vi "Teleop.vi"(10 "Match Info":T1={"Autonomous Elapsed Seconds"=0.0, "TeleOp Elapsed Seconds"=0.0, "Disabled Elapsed Seconds"=0.0, "Visited Autonomous"=FALSE, "Visited TeleOp"=FALSE, "Visited Disabled"=FALSE, "Autonomous Settings"={"Autonomous Style"=enum."Independent", "VI Refnum"=refnum}}, 11 "Call Context":T2) -> ()   [LabVIEW 2014]
doc: "This VI is called for each TeleOp packet received from the DS where the robot is not disabled. It is often used to read from the joysticks and update I/O or to update setpoints for timed control loops. It should complete and return within 20 milliseconds or it may miss DS packets."
uses:
  <vilib>/Rock Robotics/WPI/DriverStation/WPI_DriverStationDerivedRobotMode.ctl
  <vilib>/Rock Robotics/WPI/DriverStation/WPI_DriverStationMatch Info.ctl
  <vilib>/Rock Robotics/WPI/Joystick/WPI_JoystickGetSetRefNum.vi
  Robot Global Data.vi
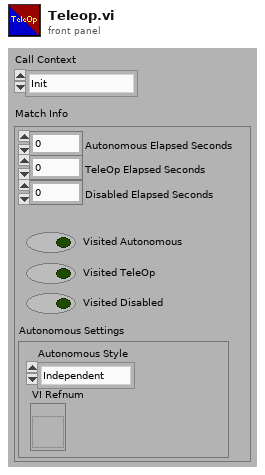
[diagram p1: front panel]
types:
  T1 = typedef "WPI_DriverStationMatch Info.ctl" = cluster{"Autonomous Elapsed Seconds":dbl, "TeleOp Elapsed Seconds":dbl, "Disabled Elapsed Seconds":dbl, "Visited Autonomous":bool, "Visited TeleOp":bool, "Visited Disabled":bool, "Autonomous Settings":cluster{"Autonomous Style":enum16{"Iterative", "Independent"}, "VI Refnum":refnum<vi>}}
  T2 = typedef "WPI_DriverStationDerivedRobotMode.ctl" = enum16{"Init", "Execute", "Stop"}
  T3 = cluster{"Initial Case":enum16{"Theta", "Arc"}, "Drive Case":enum16{"FOD", "ROD"}}
  T4 = typedef "WPI_JoystickDevRef.ctl" = cluster{"Device":T5}
  T5 = typedef "WPI_JoystickDeviceEnum.ctl" = enum16{"USB 0", "USB 1", "USB 2", "USB 3", "USB 4", "USB 5"}
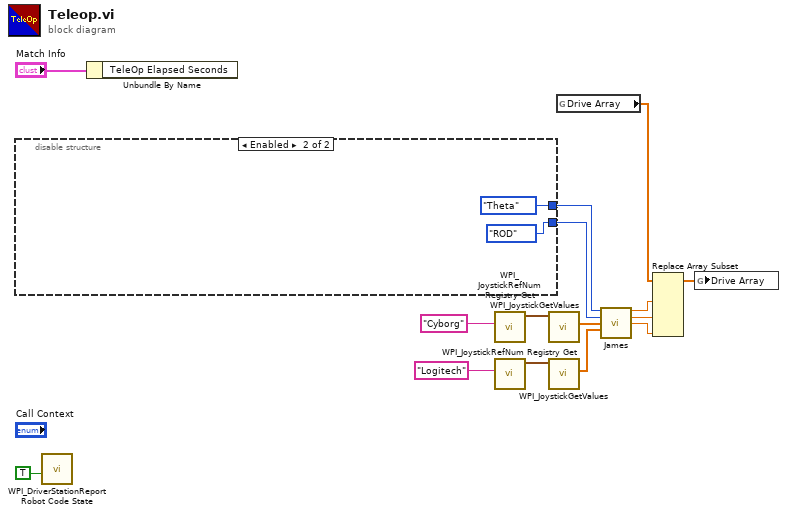
[diagram p0: block diagram]
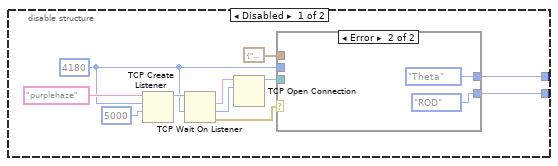
[diagram p2: hidden frame]
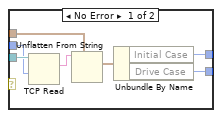
[diagram p3: hidden frame]
diagram:
  n1 = disable-structure shown="Enabled" {
    disable-tunnel: [w17 enum16{"Theta", "Arc"}."Theta" ("Initial Case")] -> w2
    disable-tunnel: [w16 enum16{"FOD", "ROD"}."ROD" ("Drive Case")] -> w1
    frame Disabled {
      w18 = u16 4180 ("remote port or service name")
      n2 = TCP Create Listener(9:5000 ("timeout ms (60000)"), 10:w18, 11:"purplehaze" ("address")) -> (3:w23:refnum<k5>)  [unwired: 2 in, 2 out]
      n3 = TCP Wait On Listener(9:w18, 11:w23) -> (0:w20:errorcluster, 1:w21:u16, 2:w22:string)  [unwired: 2 in, 2 out]
      n4 = TCP Open Connection(address=w22, remote port or service name=w21) -> (connection ID=w19:refnum<k5>)  [unwired: 3 in, 1 out]
      n5 = case shown="Error" w20 {
        tunnel: T3 {"Initial Case"=enum."Theta", "Drive Case"=enum."FOD"} -> [w33 _]
        tunnel: w19 -> [w32 _]
        tunnel: w18 -> [w30 _]
        tunnel: [w28 enum16{"Theta", "Arc"}."Theta" ("Initial Case")] -> w17
        tunnel: [w27 enum16{"FOD", "ROD"}."ROD" ("Drive Case")] -> w16
        frame No Error {
          n6 = TCP Read(connection ID=w32, 9:w30) -> (data out=w31:string)  [unwired: 3 in, 2 out]
          n7 = Unflatten From String(type=w33, binary string=w31) -> (value=w29:T3)  [unwired: 3 in, 2 out]
          n8 = Unbundle By Name(w29) -> ("Initial Case"=w28:enum16{"Theta", "Arc"}, "Drive Case"=w27:enum16{"FOD", "ROD"})
        }
        frame Error {
        }
      }
    }
    frame Enabled {
    }
  }
  n9 = call <vilib>:"WPI_DriverStationReport Robot Code State.vi"("TeleOp"=TRUE ("Autonomous")) -> ()  [unwired: 10 in, 1 out]
  n10 = Unbundle By Name("Match Info") -> ()  [unwired: 1 out]
  n11 = call <vilib>:"WPI_JoystickRefNum Registry Get.vi"("refnum name"="Cyborg") -> ("JoystickDevRef"=w11:T4)  [unwired: 9 in, 1 out]
  n12 = call <vilib>:"WPI_JoystickRefNum Registry Get.vi"("refnum name"="Logitech") -> ("JoystickDevRef"=w9:T4)  [unwired: 9 in, 1 out]
  n13 = call <vilib>:"WPI_JoystickGetValues.vi"("JoystickDevRef"=w11) -> ("Axes"=w8:dbl[])  [unwired: 6 in, 4 out]
  n14 = call <vilib>:"WPI_JoystickGetValues.vi"("JoystickDevRef"=w9) -> ("Axes"=w10:dbl[])  [unwired: 6 in, 4 out]
  n15 = global read "Robot Global Data.vi" "Drive Array"() -> (w7:dbl[])
  n16 = call "James.vi"("Initial Case"=w2, "Drive Case"=w1, "Cyborg"=w8, "Logitech"=w10) -> ("A"=w5:dbl, "B"=w4:dbl, "R"=w3:dbl)  [unwired: 9 in]
  n17 = Replace Array Subset(array=w7, new element #1=w5, new element #2=w4, new element #3=w3) -> (w6:dbl[])  [unwired: 3 in]
  n18 = global write "Robot Global Data.vi" "Drive Array"(w6) -> ()
